vi "CLD 4 Event Structure Timer-ZKL Solution.vi"() -> ()   [LabVIEW 2023]
doc: "CLD 4 Challenge Exercise"
panel:
  out "Error Out":errorcluster
  in  "Error In":errorcluster
  out "Time Has Elapsed":bool
  out "Elapsed Time":string
  in  "Auto Reset":bool=TRUE
  in  "Reset Button":bool
  in  "Stop VI":bool
  in  "Time Target (s)":dbl=4.0
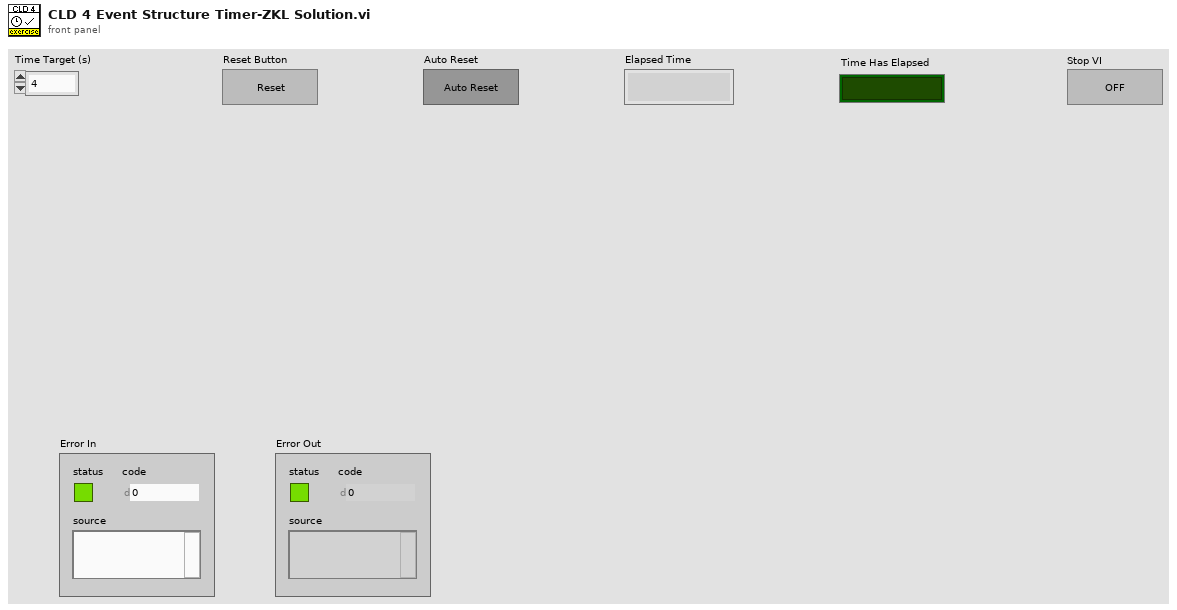
[diagram p1: front panel]
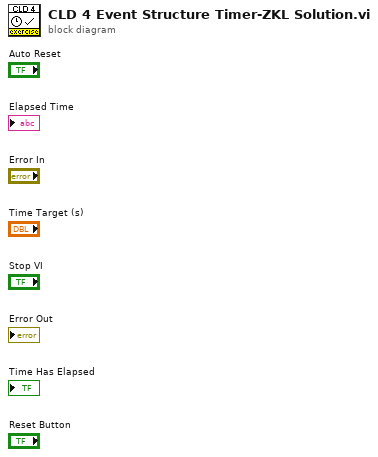
[diagram p0: block diagram]
diagram:
